vi "ReadRawAxis.vi"(8 "error in (no error)":errorcluster, 10 "Arduino Resource In":T1={"VISA resource"="", "Board Type"=enum."Uno", "Connection Type"=enum."USB / Serial", "Bytes Per Packet (15)"=15}, 11 "HMC5883L in":refnum<class "HMC5883L.lvclass">) -> (0 "error out":errorcluster, 2 "Arduino Resource out":T1={"VISA resource"="", "Board Type"=enum."Uno", "Connection Type"=enum."USB / Serial", "Bytes Per Packet (15)"=15}, 3 "HMC5883L out":refnum<class "HMC5883L.lvclass">)   [LabVIEW 2012, in "HMC5883L.lvclass"]
uses:
  HMC5883L.lvclass
  <vilib>/LabVIEW Interface for Arduino/Type Defs/Arduino Resource.ctl
  <vilib>/LabVIEW Interface for Arduino/Type Defs/Board Type.ctl
  HMC5883L.lvclass/HMC5883L.ctl
  <vilib>/LabVIEW Interface for Arduino/LabVIEW Interface for Arduino.lvlib
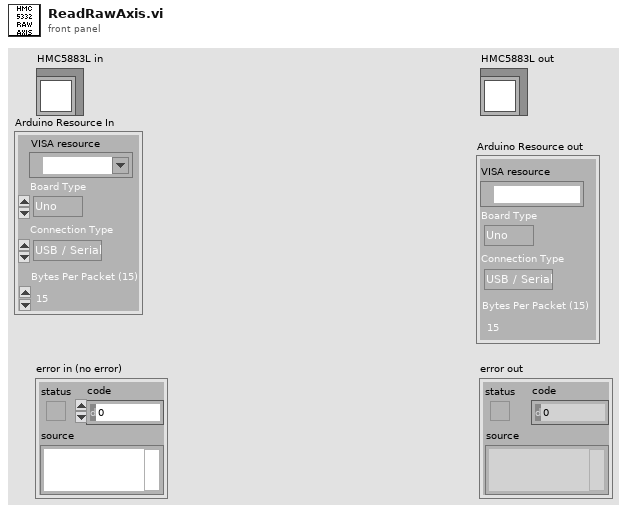
[diagram p1: front panel]
types:
  T1 = typedef "LabVIEW Interface for Arduino.lvlib/Arduino Resource.ctl" = cluster{"VISA resource":refnum<visa-resource-name>, "Board Type":T2, "Connection Type":enum8{"USB / Serial"}, "Bytes Per Packet (15)":u8}
  T2 = typedef "LabVIEW Interface for Arduino.lvlib/Board Type.ctl" = enum16{"Uno", "Dimuelanove w/Atmega 328", "Mega 2560"}
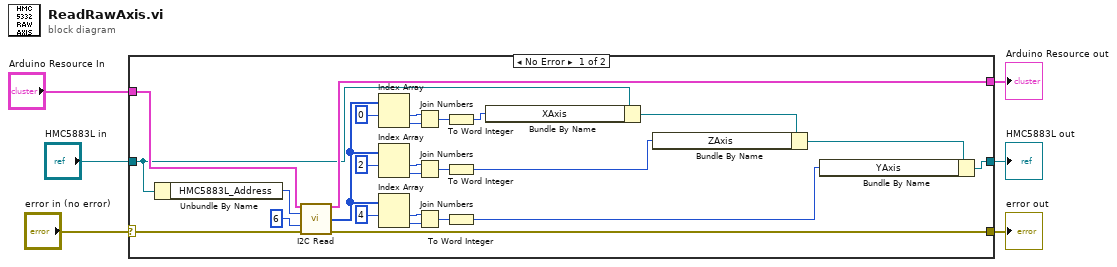
[diagram p0: block diagram]
diagram:
  n1 = case shown="No Error" "error in (no error)" {
    selector: "error in (no error)" -> [w16 w35]
    tunnel: [w15 w35] -> w5
    tunnel: [w7 w34] -> w3
    tunnel: "HMC5883L in" -> [w24 w34]
    tunnel: "Arduino Resource In" -> [w30 w33]
    tunnel: [w29 w33] -> w1
    frame No Error {
      n2 = Unbundle By Name(w24) -> ("HMC5883L_Address"=w32:u8)
      n3 = call <vilib>:"I2C Read.vi"("Arduino Resource"=w30, "Address (0)"=w32, "Bytes To Read"=u8 6, "error in"=w16) -> ("Arduino Resource"=w29:T1, "I2C Data"=w14:u8[], "error out"=w15:errorcluster)  [unwired: 9 in]
      n4 = Index Array(array=w14, index #1=0 ("index")) -> (element #1=w27:u8, element #2=w26:u8)  [unwired: 1 in]
      n5 = Index Array(array=w14, index #1=2 ("index")) -> (element #1=w20:u8, element #2=w21:u8)  [unwired: 1 in]
      n6 = Index Array(array=w14, index #1=4 ("index")) -> (element #1=w10:u8, element #2=w12:u8)  [unwired: 1 in]
      n7 = Join Numbers(hi=w27, lo=w26) -> ((hi.lo)=w25:u16)
      n8 = Join Numbers(hi=w20, lo=w21) -> ((hi.lo)=w19:u16)
      n9 = Join Numbers(hi=w10, lo=w12) -> ((hi.lo)=w11:u16)
      n10 = To Word Integer(number=w25) -> (16bit integer=w23:i16)
      n11 = To Word Integer(number=w19) -> (16bit integer=w17:i16)
      n12 = To Word Integer(number=w11) -> (16bit integer=w9:i16)
      n13 = Bundle By Name(cluster=w24, "XAxis"=w23) -> (w18:refnum<class "HMC5883L.lvclass">)
      n14 = Bundle By Name(cluster=w18, "ZAxis"=w17) -> (w8:refnum<class "HMC5883L.lvclass">)
      n15 = Bundle By Name(cluster=w8, "YAxis"=w9) -> (w7:refnum<class "HMC5883L.lvclass">)
    }
    frame Error {
    }
  }
  "error out" <- w5
  "HMC5883L out" <- w3
  "Arduino Resource out" <- w1
